vi "Building string from peak min clusters.vi"(10 "Max cluster":T1 {"Hour" format="%<%H:%M>t"}, 11 "Min Cluster":T2 {"Hour" format="%<%H:%M>t"}) -> (3 "resulting string 2":string)   [LabVIEW 2018]
panel:
  out "Numeric 2":i32
  out "hours 2":i32
  out "Min 2":i32
  out "Min":i32
  out "hours":i32
  out "Numeric":i32
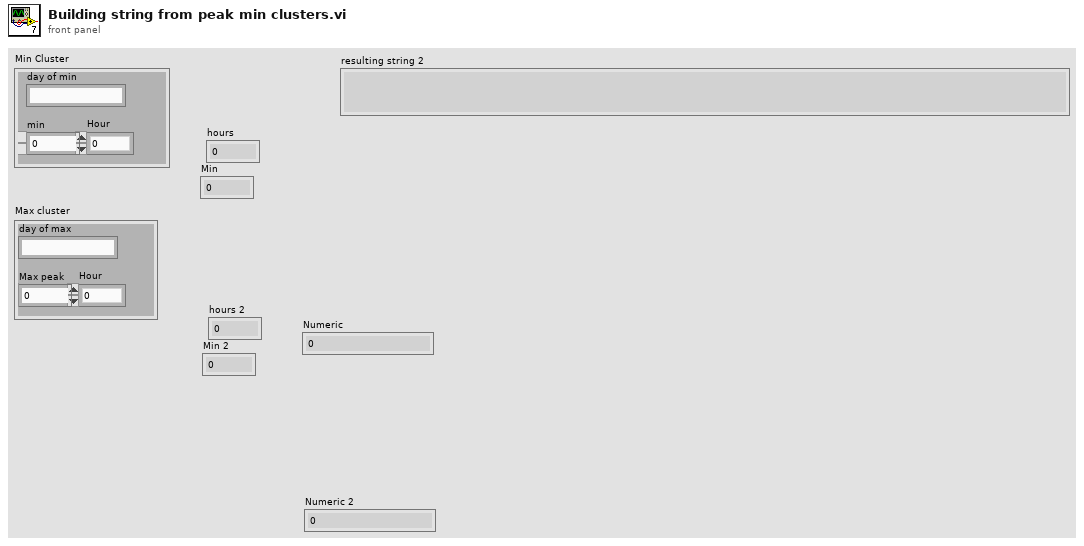
[diagram p1: front panel]
types:
  T1 = cluster{"Hour":i32, "Max peak":dbl, "day of max":string}
  T2 = cluster{"Hour":i32, "min":dbl, "day of min":string}
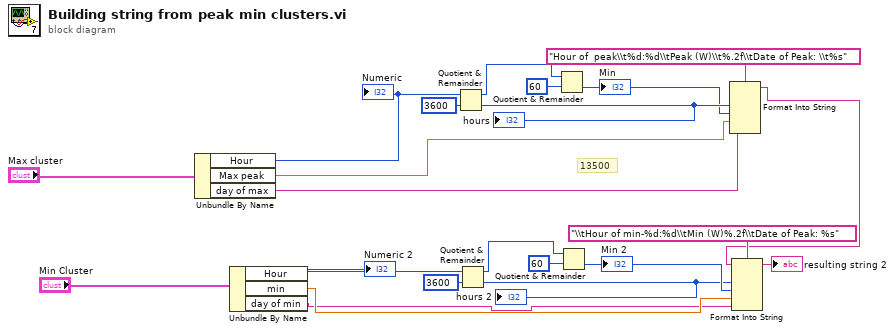
[diagram p0: block diagram]
diagram:
  # "13500"
  n1 = Unbundle By Name("Max cluster") -> ("Hour"=w14:i32, "Max peak"=w13:dbl, "day of max"=w12:string)
  "Numeric" <- w14
  n2 = Unbundle By Name("Min Cluster") -> ("Hour"=w4:i32, "min"=w3:dbl, "day of min"=w2:string)
  "Numeric 2" <- w4
  n3 = Quotient & Remainder(x=w14, y=3600) -> (x-y*floor(x/y)=w18:i32, floor(x/y)=w16:i32)
  "hours" <- w16
  n4 = Quotient & Remainder(x=w4, y=3600) -> (x-y*floor(x/y)=w8:i32, floor(x/y)=w10:i32)
  "hours 2" <- w10
  n5 = Quotient & Remainder(x=w18, y=60) -> (floor(x/y)=w15:i32)  [unwired: 1 out]
  "Min" <- w15
  n6 = Quotient & Remainder(x=w8, y=60) -> (floor(x/y)=w11:i32)  [unwired: 1 out]
  "Min 2" <- w11
  n7 = Format Into String(format string="Hour of  peak\\t%d:%d\\tPeak (W)\\t%.2f\\tDate of Peak: \\t%s", w16, w15, w13, w12) -> (resulting string=w1:string)  [unwired: 2 in, 1 out]
  n8 = Format Into String(format string="\\tHour of min-%d:%d\\tMin (W)%.2f\\tDate of Peak: %s", initial string=w1, w10, w11, w3, w2) -> (resulting string=→"resulting string 2":string)  [unwired: 1 in, 1 out]
